vi "Configure Vertical Cursors.vi"(7 "Mode (1: OFF)":i32(slide)=1, 8 "error in (no error)":errorcluster {"code" format="%.0x"}, 9 "Vertical 2 Position (0.0 Sec)":dbl format="%.2p", 10 "Vertical 1 Position (0.0 Sec)":dbl format="%.2p", 11 "VISA Resource Name":refnum<visa-resource-name>) -> (0 "error out":errorcluster {"code" format="%.0x"}, 3 "VISA Resource Name Out":refnum<visa-resource-name>)   [LabVIEW 2010, in "Tektronix TDS 3000 Series.lvlib"]
doc: "This VI configures the cursor mode and the vertical cursor positions."
uses:
  <instrlib>/Tektronix TDS 3000 Series/Tektronix TDS 3000 Series.lvlib
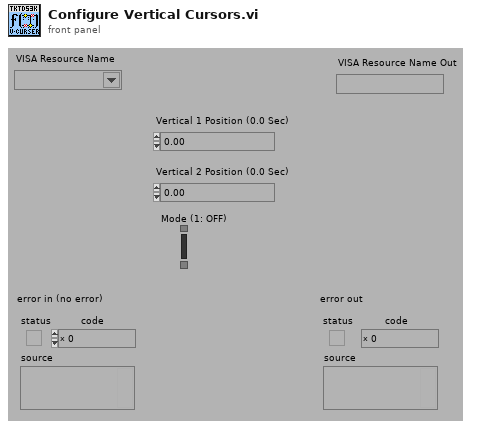
[diagram p1: front panel]
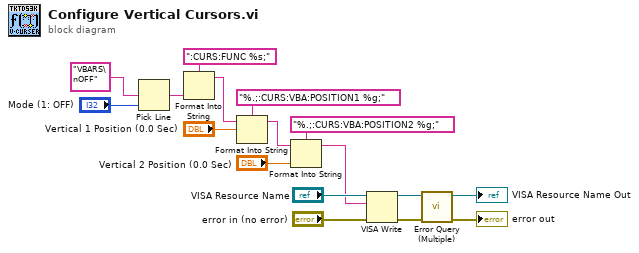
[diagram p0: block diagram]
diagram:
  n1 = Pick Line(multi-line string="VBARS\nOFF", line index="Mode (1: OFF)") -> (output string=w13:string)  [unwired: 1 in]
  n2 = Format Into String(format string=":CURS:FUNC %s;", w13) -> (resulting string=w6:string)  [unwired: 2 in, 1 out]
  n3 = Format Into String(format string="%.;:CURS:VBA:POSITION1 %g;", initial string=w6, "Vertical 1 Position (0.0 Sec)") -> (resulting string=w7:string)  [unwired: 1 in, 1 out]
  n4 = Format Into String(format string="%.;:CURS:VBA:POSITION2 %g;", initial string=w7, "Vertical 2 Position (0.0 Sec)") -> (resulting string=w5:string)  [unwired: 1 in, 1 out]
  n5 = VISA Write(VISA resource name="VISA Resource Name", write buffer=w5, error in (no error)="error in (no error)") -> (VISA resource name out=w4:refnum<visa-resource-name>, error out=w3:errorcluster)  [unwired: 1 out]
  n6 = call <instrlib>:"Error Query (Multiple).vi"("error in (no error)"=w3, "VISA Resource Name"=w4) -> ("error out"=→"error out":errorcluster, "VISA Resource Name Out"=→"VISA Resource Name Out":refnum<visa-resource-name>)  [unwired: 6 in, 2 out]
